vi "未命名 3.vi"   [LabVIEW 2020]
uses:
  <vilib>/eio/EIONode/EIONode.xnode
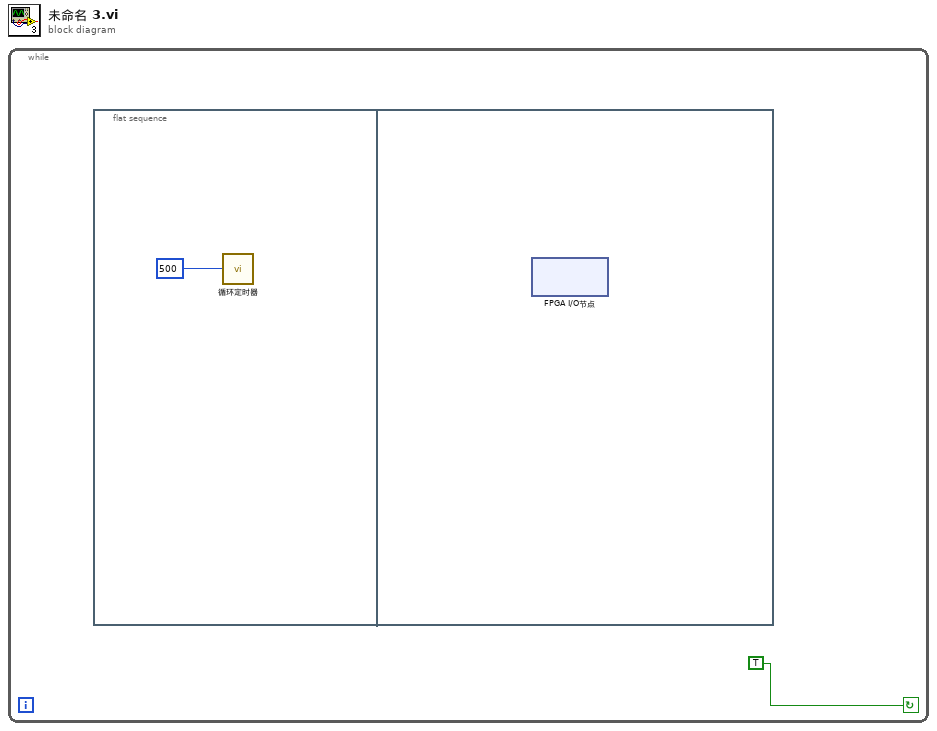
[diagram p0: block diagram]
diagram:
  n1 = while {
    stop <- TRUE continue-if-true
    n2 = flat-sequence {
      frame #0 {
        n3 = call "循环定时器"("Count(uSec)"=i16 500) -> ()  [unwired: 1 out]
      }
      frame #1 {
        n4 = xnode "FPGA I/O节点"() -> ()  [unwired: 1 in, 2 out]
      }
    }
  }
